vi "Read IPS Level.vi"(8 "error in (no error)":errorcluster, 11 "Instrument.Oxford1820 in":refnum<class "Instrument.Oxford1820.lvclass">) -> (0 "error out":errorcluster, 1 "N2 Level (%)":dbl, 2 "He Level (%)":dbl, 3 "Instrument.Oxford1820 out":refnum<class "Instrument.Oxford1820.lvclass">)   [LabVIEW 2019, in "Instrument.Oxford1820.lvclass"]
uses:
  Instrument.Oxford1820.lvclass
  Instrument.Oxford1820.lvclass/Instrument.Oxford1820.ctl
  <instrlib>/Mercury iXX/Public/Libraries/Level Meter/Open/Open Level Meter Device.vi
  <instrlib>/Mercury iXX/Public/Libraries/Level Meter/Signals/Read/Probe Level Helium (Read).vi
  <instrlib>/Mercury iXX/Public/Libraries/Level Meter/Signals/Read/Probe Level Nitrogen (Read).vi
  <instrlib>/Mercury iXX/Mercury iXX.lvlib
  <instrlib>/Mercury iXX/Public/Libraries/Level Meter.lvlib
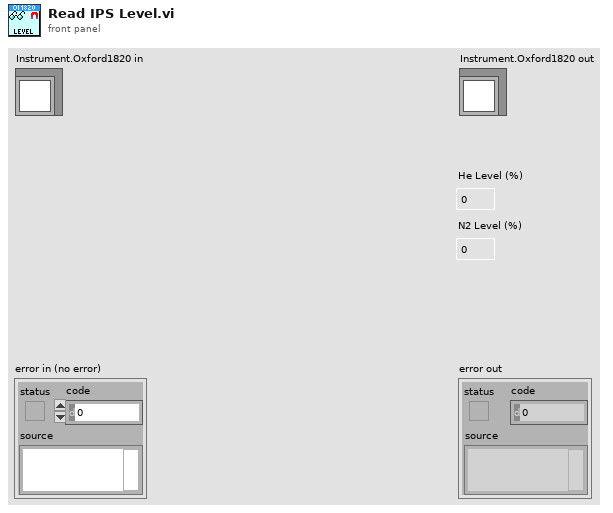
[diagram p1: front panel]
types:
  T1 = typedef "Mercury iXX.lvlib/Mercury Reference.ctl" = cluster{"Comms":refnum<visa-resource-name>, "Device ID":string[], "Comms Layer":T2, "Command":string, "Query reference":T3}
  T2 = typedef "Mercury iXX.lvlib/Comms Transport Layer.ctl" = enum16{"Ethernet TCP/IP", "USB", "ISOBus - RS-232", "GPIB"}
  T3 = typedef "Mercury iXX.lvlib/Query Dynamic Reference.ctl" = refnum<vi>
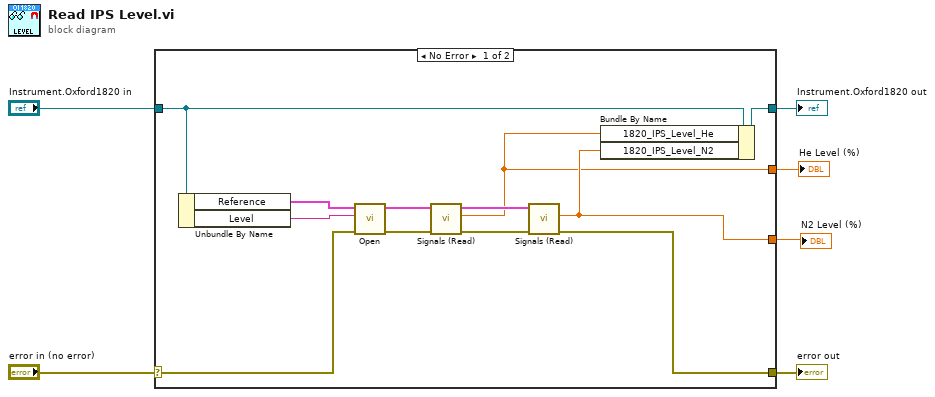
[diagram p0: block diagram]
diagram:
  n1 = case shown="No Error" "error in (no error)" {
    selector: "error in (no error)" -> [w14 w20]
    tunnel: [w11 w20] -> w5
    tunnel: [w10 w19] -> w3
    tunnel: "Instrument.Oxford1820 in" -> [w9 w19]
    tunnel: [w7 _] -> w2
    tunnel: [w8 _] -> w1
    frame No Error {
      n2 = Unbundle By Name(w9) -> ("Reference"=w15:T1, "Level"=w16:string)
      n3 = call-poly <instrlib>:"Open.vi"("error in (no error)"=w14, "Device Identifier"=w16, "Mercury Reference In"=w15) -> ("error out"=w18:errorcluster, "Mercury Reference Out"=w17:T1)  [unwired: 7 out]
      n4 = call-poly <instrlib>:"Signals (Read).vi"("error in"=w18, "Mercury Reference In"=w17) -> ("error out"=w13:errorcluster, "Level"=w7:dbl, "Mercury Reference Out"=w12:T1)  [unwired: 1 in, 6 out]
      n5 = call-poly <instrlib>:"Signals (Read).vi"("error in"=w13, "Mercury Reference In"=w12) -> ("error out"=w11:errorcluster, "Level"=w8:dbl)  [unwired: 1 in, 7 out]
      n6 = Bundle By Name(cluster=w9, "1820_IPS_Level_He"=w7, "1820_IPS_Level_N2"=w8) -> (w10:refnum<class "Instrument.Oxford1820.lvclass">)
    }
    frame Error {
    }
  }
  "error out" <- w5
  "Instrument.Oxford1820 out" <- w3
  "He Level (%)" <- w2
  "N2 Level (%)" <- w1
